vi "Global 3.vi"() -> ()   [LabVIEW 2012]
panel:
  in  "Stop Program and Write to File":bool
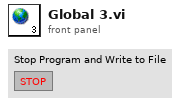
[diagram p1: front panel]
diagram:
